vi "SetRooms.vi"(0 "House in":refnum<class "House.lvclass">, 5 "Rooms":refnum<class "Room.lvclass">[](array[class]), 11 "error in (no error)":errorcluster) -> (4 "House out":refnum<class "House.lvclass">, 15 "error out":errorcluster)   [LabVIEW 2019, in "House.lvclass"]
uses:
  House.lvclass
  Room.lvclass
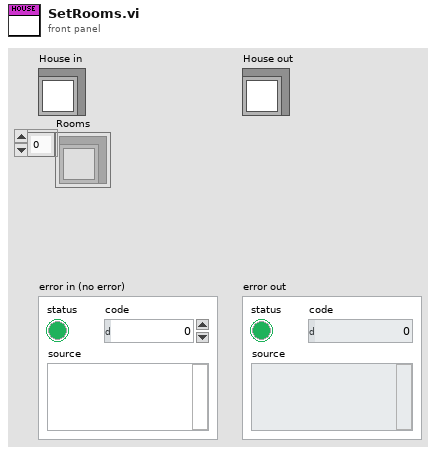
[diagram p1: front panel]
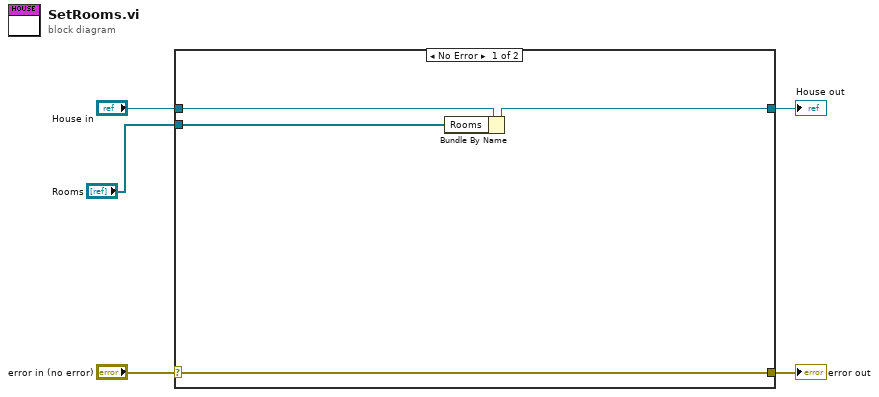
[diagram p0: block diagram]
diagram:
  n1 = case shown="No Error" "error in (no error)" {
    selector: "error in (no error)" -> [w9 w11]
    tunnel: [w9 w11] -> w2
    tunnel: [w7 w10] -> w4
    tunnel: "House in" -> [w8 w10]
    tunnel: "Rooms" -> [w6 _]
    frame No Error {
      n2 = Bundle By Name(cluster=w8, "Rooms"=w6) -> (w7:refnum<class "House.lvclass">)
    }
    frame Error {
    }
  }
  "House out" <- w4
  "error out" <- w2
